vi "AngleBetweenPoints.vi"(10 "Point 2":T1 {"North" format="%#_10f"; "East" format="%#_8f"}, 11 "Point 1":T1 {"North" format="%#_10f"; "East" format="%#_8f"}) -> (2 "Angle":dbl)   [LabVIEW 2013]
doc: "Takes in two UTM points and calculates the angle between them. The angle is in the standard reference frame."
uses:
  Data/TypeDefs/UTM Location.ctl
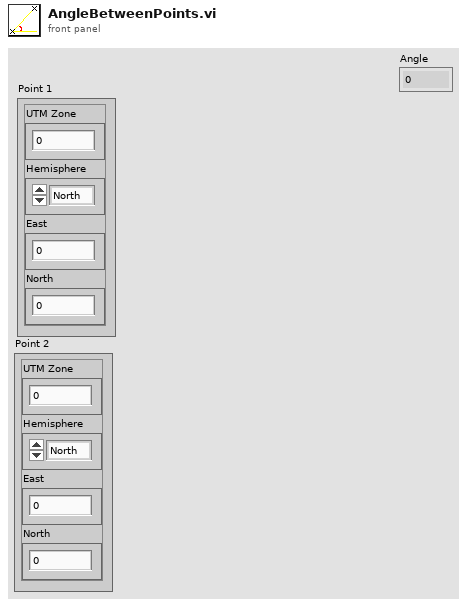
[diagram p1: front panel]
types:
  T1 = typedef "UTM Location.ctl" = cluster{"UTM Zone":dbl, "Hemisphere":enum16{"North", "South"}, "East":dbl, "North":dbl}
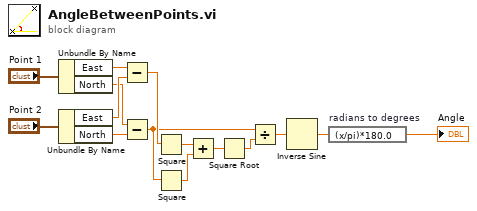
[diagram p0: block diagram]
diagram:
  n1 = Unbundle By Name("Point 1") -> ("East"=w13:dbl, "North"=w10:dbl)
  n2 = Unbundle By Name("Point 2") -> ("East"=w12:dbl, "North"=w11:dbl)
  n3 = Subtract(x=w13, y=w12) -> (x-y=w9:dbl)
  n4 = Subtract(x=w10, y=w11) -> (x-y=w4:dbl)
  n5 = Square(x=w9) -> (x^2=w8:dbl)
  n6 = Square(x=w4) -> (x^2=w7:dbl)
  n7 = Add(x=w8, y=w7) -> (x+y=w6:dbl)
  n8 = Square Root(x=w6) -> (sqrt(x)=w5:dbl)
  n9 = Divide(x=w4, y=w5) -> (x/y=w3:dbl)
  n10 = Inverse Sine(1:w3) -> (0:w2:dbl)
  n11 = expression code="(x/pi)*180.0" "radians to degrees"(w2) -> (→"Angle":dbl)
